vi "ExecuteToolMenuCommand.vi"(0 "reference in":refnum<class "DqmhModuleDiagramGraph.lvclass">, 1 "MenuItemTag":string, 2 "selected":T1, 3 "selectedEdge":refnum<class "AbstractEdge.lvclass">, 4 "SelectedNodes":refnum<class "AbstractNode.lvclass">[](array[class]), 5 "error in (no error)":errorcluster) -> (14 "reference out":refnum<class "DqmhModuleDiagramGraph.lvclass">, 15 "Handled":bool, 19 "error out":errorcluster)   [LabVIEW 2014, in "DqmhModuleDiagramGraph.lvclass"]
uses:
  <resource>/Framework/Providers/Open_GDS/UML/DqmhModuleDiagramGraph_class/DqmhModuleDiagramGraph.lvclass
  <resource>/Framework/Providers/Open_GDS/UML/AbstractEdge_class/AbstractEdge.lvclass
  <resource>/Framework/Providers/Open_GDS/UML/AbstractNode_class/AbstractNode.lvclass
  <resource>/Framework/Providers/Open_GDS/UML/UMLEditor/UMLEditor tooltype.ctl
  <resource>/Framework/Providers/Open_GDS/UML/DQMHModuleNode_class/DQMHModuleNode.lvclass
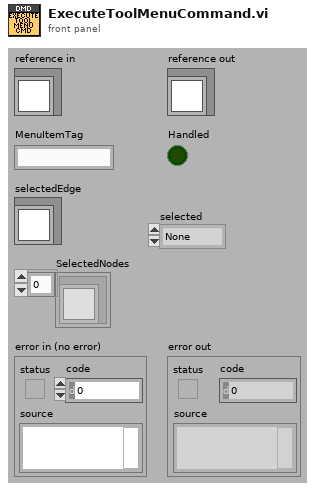
[diagram p1: front panel]
types:
  T1 = typedef "UMLEditor tooltype.ctl" = enum16{"None", "Node", "Edge"}
  T2 = cluster{string, string, "short cut out":cluster{"include Shift key?":bool, "include Ctrl key? ":bool, "shortcut key":string}}[]
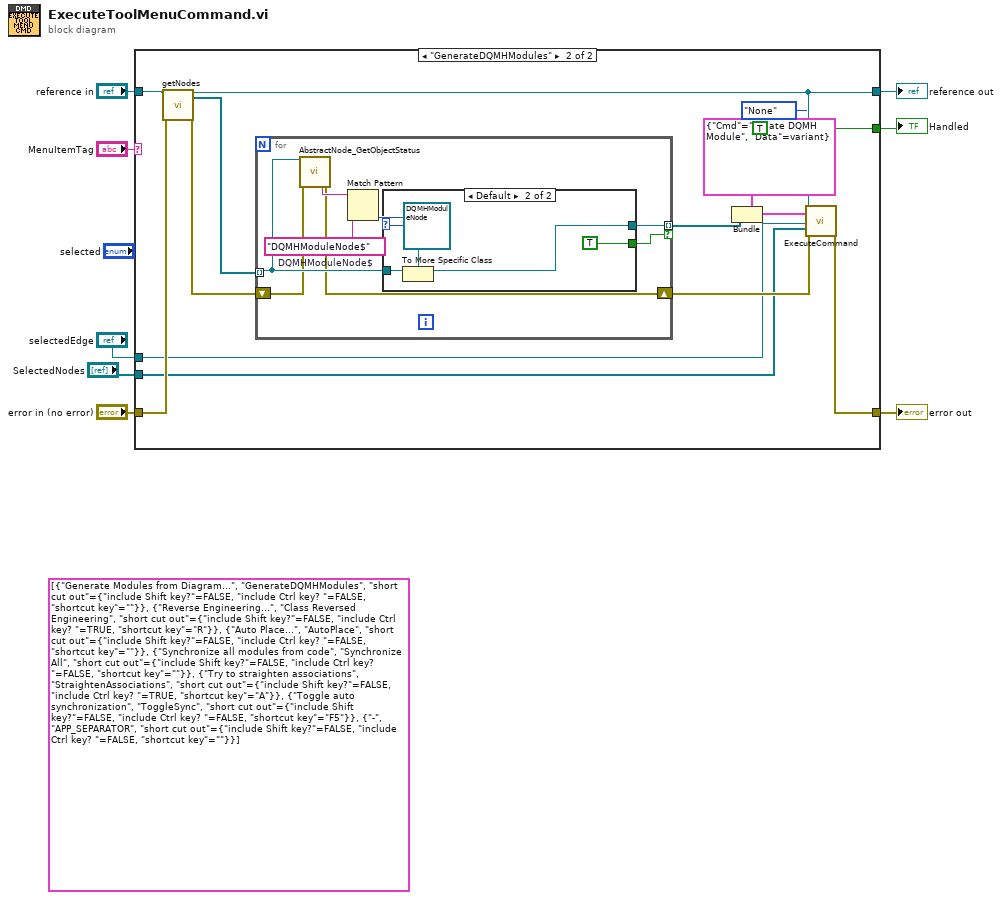
[diagram p0: block diagram]
diagram:
  (unwired) T2 [{"Generate Modules from Diagram...", "GenerateDQMHModules", "short cut out"={"include Shift key?"=FALSE, "include Ctrl key? "=FALSE, "shortcut key"=""}}, {"Reverse Engineering...", "Class Reversed Engineering", "short cut out"={"include Shift key?"=FALSE, "include Ctrl key? "=TRUE, "shortcut key"="R"}}, {"Auto Place...", "AutoPlace", "short cut out"={"include Shift key?"=FALSE, "include Ctrl key? "=FALSE, "shortcut key"=""}}, {"Synchronize all modules from code", "Synchronize All", "short cut out"={"include Shift key?"=FALSE, "include Ctrl key? "=FALSE, "shortcut key"=""}}, {"Try to straighten associations", "StraightenAssociations", "short cut out"={"include Shift key?"=FALSE, "include Ctrl key? "=TRUE, "shortcut key"="A"}}, {"Toggle auto synchronization", "ToggleSync", "short cut out"={"include Shift key?"=FALSE, "include Ctrl key? "=FALSE, "shortcut key"="F5"}}, {"-", "APP_SEPARATOR", "short cut out"={"include Shift key?"=FALSE, "include Ctrl key? "=FALSE, "shortcut key"=""}}]
  n1 = case shown="\"GenerateDQMHModules\"" "MenuItemTag" {
    tunnel: [w9 w14] -> w7
    tunnel: [w10 w16] -> w5
    tunnel: "reference in" -> [w10 w22]
    tunnel: "error in (no error)" -> [w9 w23]
    tunnel: [_ TRUE ("include Ctrl key?")] -> w3
    tunnel: "SelectedNodes" -> [_ w13]
    tunnel: "selectedEdge" -> [_ w12]
    frame Default {
    }
    frame "GenerateDQMHModules" {
      n2 = call-dynamic "getNodes.vi"("reference"=w22, "error in (no error)"=w23) -> ("reference out"=w16:refnum<class "DqmhModuleDiagramGraph.lvclass">, "nodes"=w21:refnum<class "AbstractNode.lvclass">[], "error out"=w20:errorcluster)  [unwired: 15 in]
      n3 = for {
        tunnel: w21 -> [w29] mode=indexing
        shift-right: [w26] -> w15
        shift-left: w20 -> [w27]
        tunnel: [w28] -> w18 mode=indexing if=w25
        w31 = "DQMHModuleNode$"  # DQMHModuleNode$
        n4 = call <resource>:"AbstractNode_GetObjectStatus.vi"("reference in"=w29, "error in (no error)"=w27) -> ("Class name"=w32:string, "error out"=w26:errorcluster)  [unwired: 16 out]
        n5 = Match Pattern(string=w32, regular expression=w31) -> (offset past match=w30:i32)  [unwired: 4 out]
        n6 = case shown="Default" w30 {
          tunnel: w29 -> [_ w36]
          tunnel: [_ w34] -> w28
          tunnel: [_ TRUE] -> w25
          frame -1 {
          }
          frame Default {
            n7 = To More Specific Class(target class=refnum<class "DQMHModuleNode.lvclass"> refnum ("DQMHModuleNode"), reference=w36) -> (specific class reference=w34:refnum<class "DQMHModuleNode.lvclass">)  [unwired: 1 in, 1 out]
          }
        }
      }
      n8 = Bundle(cluster=cluster{"Cmd":string, "Data":variant} {"Cmd"="Create DQMH Module", "Data"=variant} ("FlattenCommandSettings"), "Data"=w18) -> (w17:cluster{"Cmd":string, "Data":variant})  [unwired: 1 in]
      n9 = call-dynamic "ExecuteCommand.vi"("reference in"=w16, "CommandData"=w17, "toolType"=UMLEditor_tooltype."None" ("selected"), "selectedEdge"=w12, "SelectedNodes"=w13, "error in (no error)"=w15) -> ("error out"=w14:errorcluster)  [unwired: 11 in, 2 out]
    }
  }
  "error out" <- w7
  "reference out" <- w5
  "Handled" <- w3
